vi "Run_2_of_6_Tests.vi"() -> ()   [LabVIEW 2019]
uses:
  <vilib>/Rock Robotics/WPI/ThirdParty/JAS_Junk/TrajLib/Trajectory_Library.lvlib
panel:
  out "String":string
  out "Flywheel Simulation":bool
  out "Matrix":bool
  out "PID":bool
  out "Math Utils":bool
  out "Linear Filter":bool
  out "Linear System Loop":bool
  out "All Tests Finished":bool
  out "Holonomic Drive Ctrl":bool
  out "Linear Plant Inv FF":bool
  out "Numerical Jacobian":bool
  out "Merwe Scaled Sigma Pts":bool
  out "Numerical Integration":bool
  out "Median Filter":bool
  out "Linear System ID":bool
  out "Kalman filter":bool
  out "PID Input / Output":bool
  out "Linear Quadradtic Regulator":bool
  # "FORMAL TRAJECTORY / CONTROL LIBRARY TEST PROCEDURE"
  # "FUNCTION NOT\nIMPLEMENTED"
  # "Extended Kalman Filter"
  # "Mech Drive Kinematics"
  # "Mech Drive Odometry"
  # "Mech Drive Pose Est"
  # "FUNCTION NOT\nIMPLEMENTED"
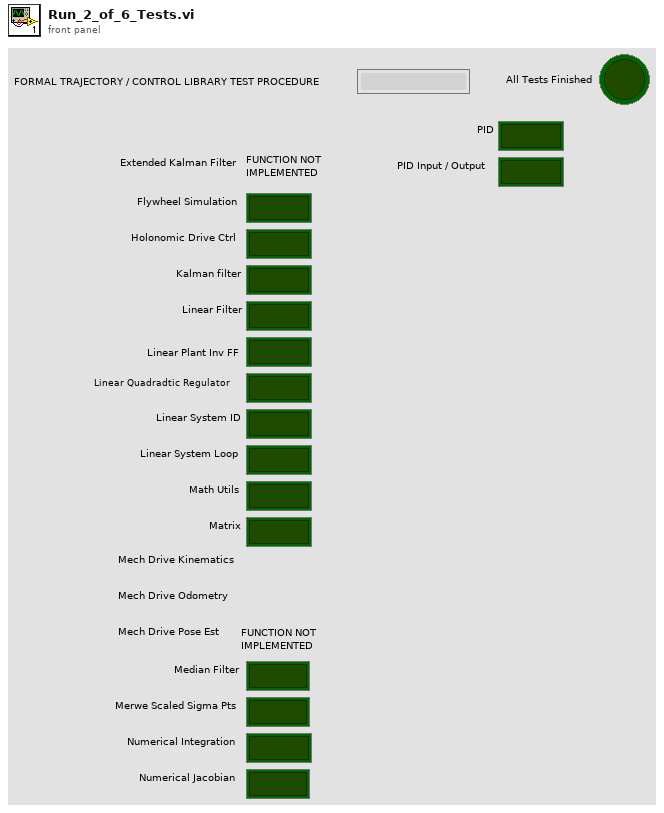
[diagram p1: front panel]
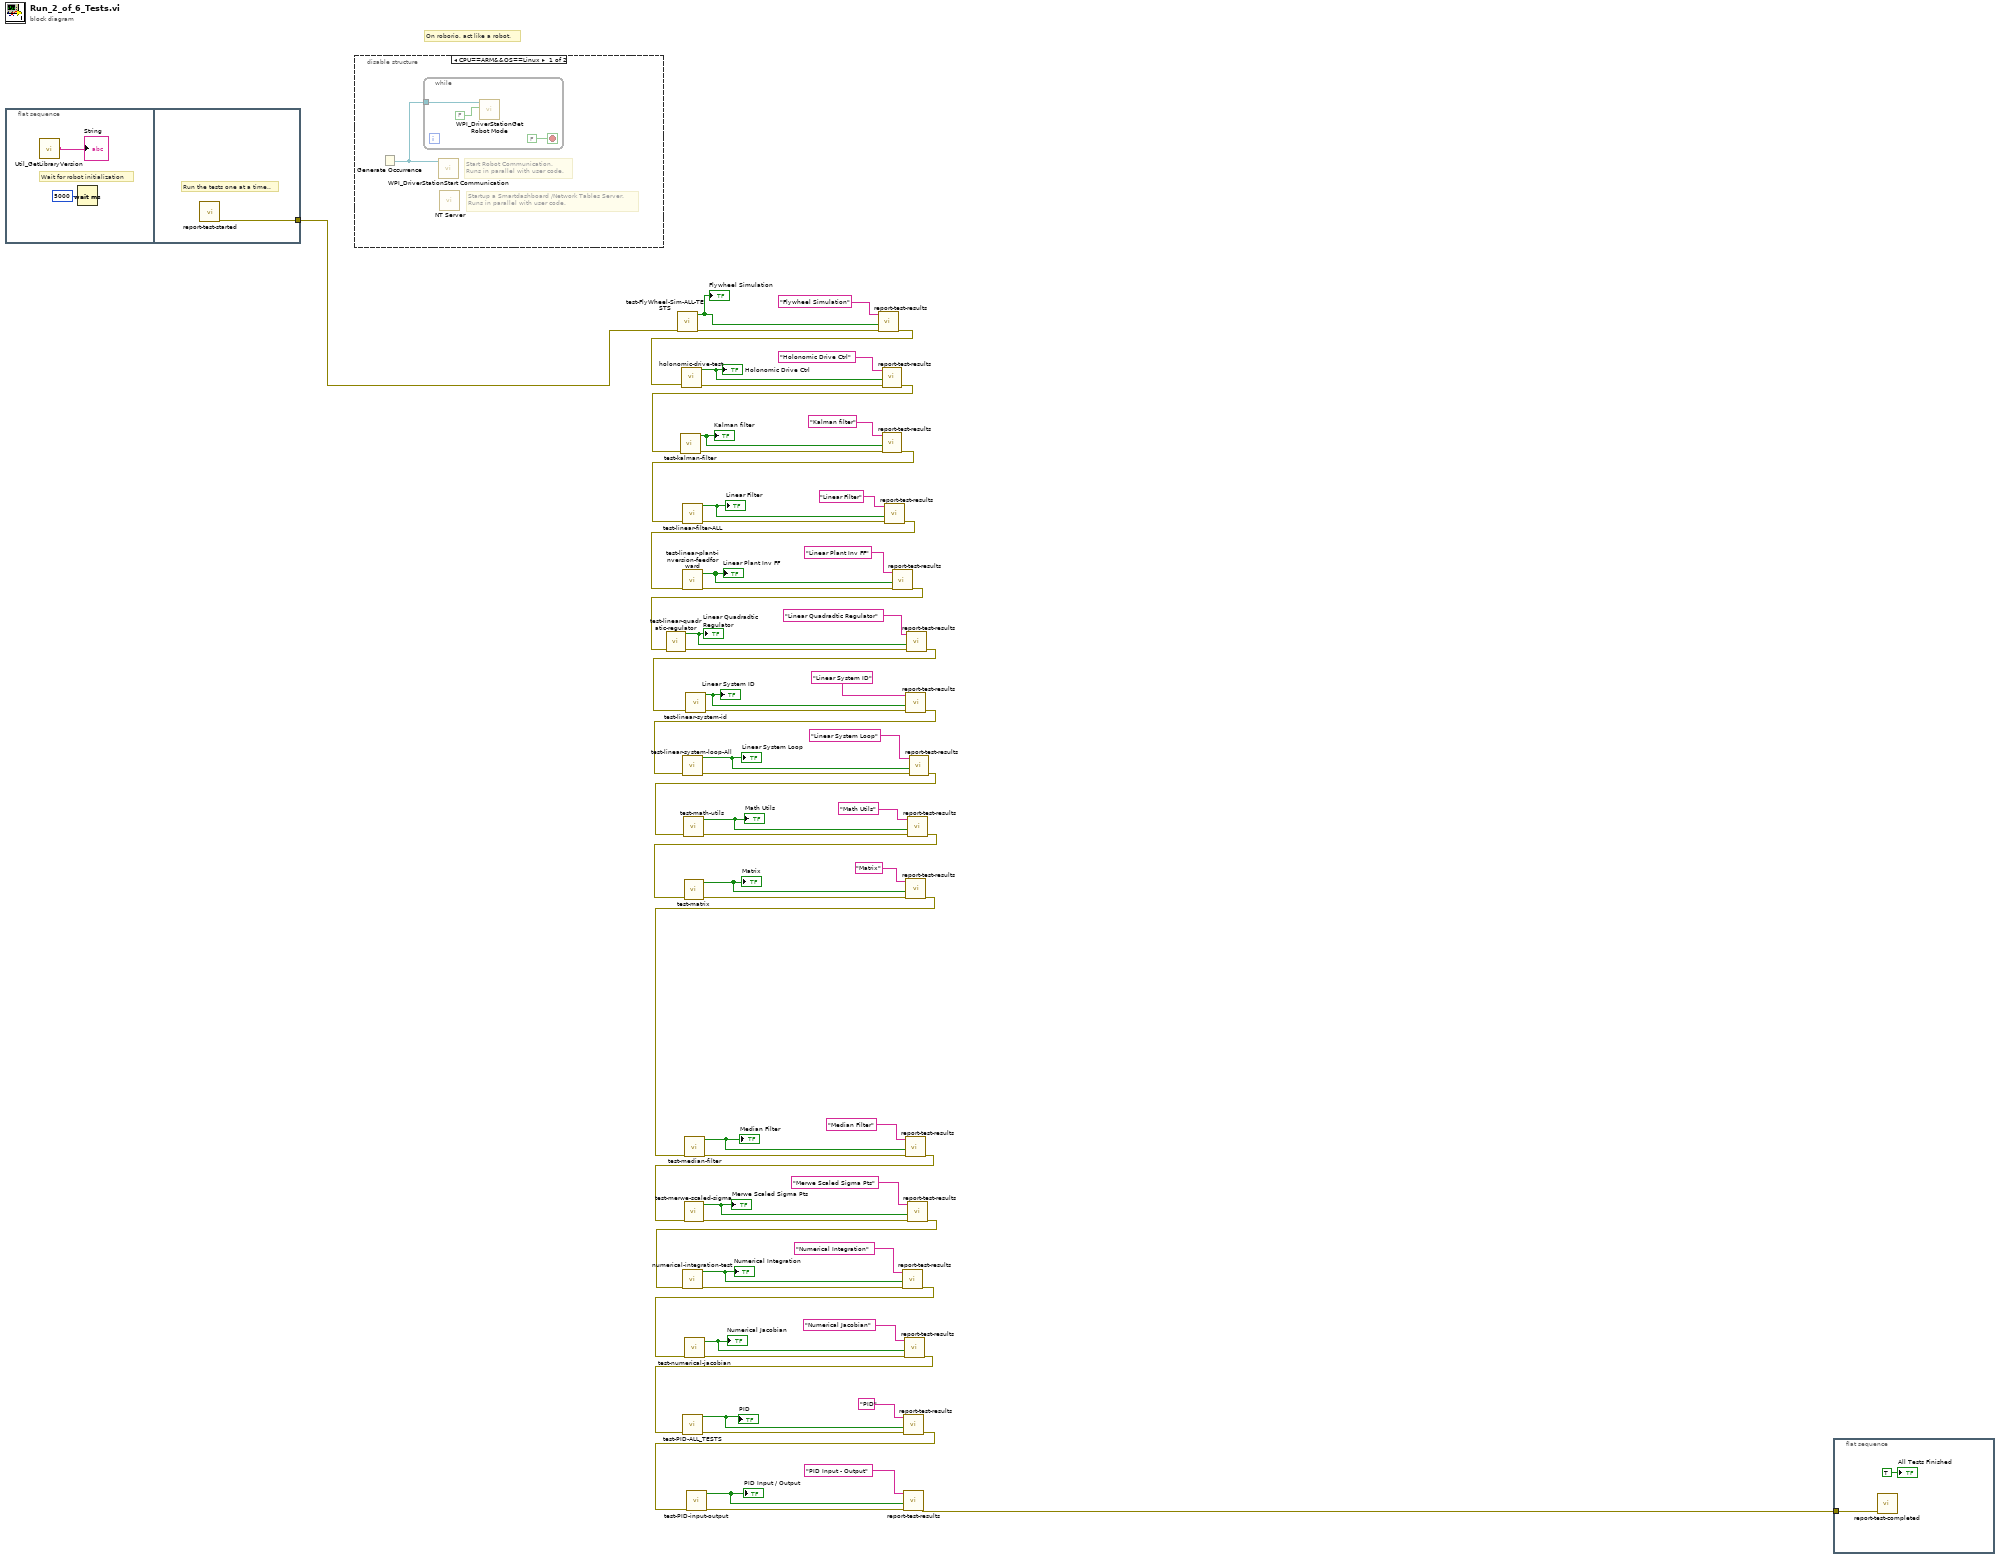
[diagram p0: block diagram]
diagram:
  # "On roborio, act like a robot."
  n1 = flat-sequence {
    tunnel: [w68] -> w3
    frame #0 {
      # "Wait for robot initialization"
      n2 = call <vilib>:"Util_GetLibraryVersion.vi"() -> ("TrajLibVersion"=→"String":string)  [unwired: 11 in]
      n3 = Wait (ms)(milliseconds to wait=u32 5000) -> ()  [unwired: 1 out]
    }
    frame #1 {
      # "Run the tests one at a time.."
      n4 = call "report-test-started.vi"() -> ("error out"=w68:errorcluster)  [unwired: 11 in]
    }
  }
  n5 = disable-structure shown="CPU==ARM&&OS==Linux" {
    frame condition #0 {
      # "Startup a Smartdashboard /Network Tables Server.\nRuns in parallel with user code."
      # "Start Robot Communication.\nRuns in parallel with user code."
      n6 = Generate Occurrence() -> (w69:refnum<k4>)
      n7 = while {
        tunnel: w69 -> [w72]
        stop <- FALSE stop-if-true
        n8 = call <vilib>:"WPI_DriverStationGet Robot Mode.vi"("Finish"=FALSE, "DS Occurrence"=w72) -> ()  [unwired: 10 out]
      }
      n9 = call <vilib>:"WPI_DriverStationStart Communication.vi"("occurrence"=w69) -> ()  [unwired: 2 in, 9 out]
      n10 = call <vilib>:"NT Server.vi"() -> ()  [unwired: 12 in]
    }
    frame condition #1 (active) {
    }
  }
  n11 = call "test-FlyWheel-Sim-ALL-TESTS.vi"("error in (no error)"=w3) -> ("error out"=w4:errorcluster, "All Passed"=w1:bool)  [unwired: 9 in]
  "Flywheel Simulation" <- w1
  n12 = call "report-test-results.vi"("error in (no error)"=w4, "TestPassed"=w1, "Test Name"="Flywheel Simulation") -> ("error out"=w2:errorcluster)  [unwired: 8 in]
  n13 = call "holonomic-drive-test.vi"("error in (no error)"=w2) -> ("error out"=w35:errorcluster, "ALL TESTS PASSED"=w63:bool)  [unwired: 9 in]
  "Holonomic Drive Ctrl" <- w63
  n14 = call "report-test-results.vi"("error in (no error)"=w35, "TestPassed"=w63, "Test Name"="Holonomic Drive Ctrl") -> ("error out"=w34:errorcluster)  [unwired: 8 in]
  n15 = call "test-kalman-filter.vi"("error in (no error)"=w34) -> ("error out"=w33:errorcluster, "ALL TESTS PASSED"=w62:bool)  [unwired: 9 in]
  "Kalman filter" <- w62
  n16 = call "report-test-results.vi"("error in (no error)"=w33, "TestPassed"=w62, "Test Name"="Kalman filter") -> ("error out"=w32:errorcluster)  [unwired: 8 in]
  n17 = call "test-linear-filter-ALL.vi"("error in (no error)"=w32) -> ("error out"=w30:errorcluster, "ALL TESTS GOOD"=w53:bool)  [unwired: 9 in]
  "Linear Filter" <- w53
  n18 = call "report-test-results.vi"("error in (no error)"=w30, "TestPassed"=w53, "Test Name"="Linear Filter") -> ("error out"=w29:errorcluster)  [unwired: 8 in]
  n19 = call "test-linear-plant-inversion-feedforward.vi"("error in (no error)"=w29) -> ("error out"=w28:errorcluster, "All Tests Passed"=w52:bool)  [unwired: 9 in]
  "Linear Plant Inv FF" <- w52
  n20 = call "report-test-results.vi"("error in (no error)"=w28, "TestPassed"=w52, "Test Name"="Linear Plant Inv FF") -> ("error out"=w27:errorcluster)  [unwired: 8 in]
  n21 = call "test-linear-quadratic-regulator.vi"("error in (no error)"=w27) -> ("error out"=w26:errorcluster, "ALL TESTS GOOD"=w51:bool)  [unwired: 9 in]
  "Linear Quadradtic Regulator" <- w51
  n22 = call "report-test-results.vi"("error in (no error)"=w26, "TestPassed"=w51, "Test Name"="Linear Quadradtic Regulator") -> ("error out"=w25:errorcluster)  [unwired: 8 in]
  n23 = call "test-linear-system-id.vi"("error in (no error)"=w25) -> ("error out"=w24:errorcluster, "All tests passed"=w50:bool)  [unwired: 9 in]
  "Linear System ID" <- w50
  n24 = call "report-test-results.vi"("error in (no error)"=w24, "TestPassed"=w50, "Test Name"="Linear System ID") -> ("error out"=w16:errorcluster)  [unwired: 8 in]
  n25 = call "test-linear-system-loop-All.vi"("error in (no error)"=w16) -> ("error out"=w17:errorcluster, "ALL TEsts Passed"=w49:bool)  [unwired: 9 in]
  "Linear System Loop" <- w49
  n26 = call "report-test-results.vi"("error in (no error)"=w17, "TestPassed"=w49, "Test Name"="Linear System Loop") -> ("error out"=w15:errorcluster)  [unwired: 8 in]
  n27 = call "test-math-utils.vi"("error in (no error)"=w15) -> ("error out"=w14:errorcluster, "ALL TESTS PASSED"=w48:bool)  [unwired: 9 in]
  "Math Utils" <- w48
  n28 = call "report-test-results.vi"("error in (no error)"=w14, "TestPassed"=w48, "Test Name"="Math Utils") -> ("error out"=w13:errorcluster)  [unwired: 8 in]
  n29 = call "test-matrix.vi"("error in (no error)"=w13) -> ("error out"=w18:errorcluster, "All Tests\nPassed"=w47:bool)  [unwired: 9 in]
  "Matrix" <- w47
  n30 = call "report-test-results.vi"("error in (no error)"=w18, "TestPassed"=w47, "Test Name"="Matrix") -> ("error out"=w12:errorcluster)  [unwired: 8 in]
  n31 = call "test-median-filter.vi"("error in (no error)"=w12) -> ("error out"=w19:errorcluster, "ALL TESTS PASSED"=w46:bool)  [unwired: 9 in]
  "Median Filter" <- w46
  n32 = call "report-test-results.vi"("error in (no error)"=w19, "TestPassed"=w46, "Test Name"="Median Filter") -> ("error out"=w11:errorcluster)  [unwired: 8 in]
  n33 = call "test-merwe-scaled-sigma.vi"("error in (no error)"=w11) -> ("error out"=w20:errorcluster, "All Tests Passed"=w36:bool)  [unwired: 9 in]
  "Merwe Scaled Sigma Pts" <- w36
  n34 = call "report-test-results.vi"("error in (no error)"=w20, "TestPassed"=w36, "Test Name"="Merwe Scaled Sigma Pts") -> ("error out"=w10:errorcluster)  [unwired: 8 in]
  n35 = call "numerical-integration-test.vi"("error in (no error)"=w10) -> ("error out"=w21:errorcluster, "All passed"=w37:bool)  [unwired: 9 in]
  "Numerical Integration" <- w37
  n36 = call "report-test-results.vi"("error in (no error)"=w21, "TestPassed"=w37, "Test Name"="Numerical Integration") -> ("error out"=w9:errorcluster)  [unwired: 8 in]
  n37 = call "test-numerical-jacobian.vi"("error in (no error)"=w9) -> ("error out"=w22:errorcluster, "ALL Tests Passed"=w38:bool)  [unwired: 9 in]
  "Numerical Jacobian" <- w38
  n38 = call "report-test-results.vi"("error in (no error)"=w22, "TestPassed"=w38, "Test Name"="Numerical Jacobian") -> ("error out"=w8:errorcluster)  [unwired: 8 in]
  n39 = call "test-PID-ALL_TESTS.vi"("error in (no error)"=w8) -> ("error out"=w23:errorcluster, "All Passed"=w39:bool)  [unwired: 9 in]
  "PID" <- w39
  n40 = call "report-test-results.vi"("error in (no error)"=w23, "TestPassed"=w39, "Test Name"="PID") -> ("error out"=w7:errorcluster)  [unwired: 8 in]
  n41 = call "test-PID-input-output.vi"("error in (no error)"=w7) -> ("error out"=w31:errorcluster, "All Passed"=w40:bool)  [unwired: 9 in]
  "PID Input / Output" <- w40
  n42 = call "report-test-results.vi"("error in (no error)"=w31, "TestPassed"=w40, "Test Name"="PID Input - Output") -> ("error out"=w6:errorcluster)  [unwired: 8 in]
  n43 = flat-sequence {
    tunnel: w6 -> [w73]
    frame #0 {
      n44 = call "report-test-completed.vi"("error in (no error)"=w73) -> ()  [unwired: 10 in, 1 out]
      "All Tests Finished" <- TRUE ("All Tests Finished")
    }
  }
